vi "Mode 2 - 2D FF AUT Test.vi"() -> (2 "Mode2 Test Properties":T1, 3 "Cancelled?":bool)   [LabVIEW 2019]
doc: "Use this template to create a dialog box with event handling."
uses:
  Mode2TestProperties.ctl
  Classes/Sequence/SequenceSubvis/RF Direction.ctl
panel:
  in  "VNA Calibration File":path
  in  "Number of FF Points":i32
  in  "dPhi (deg)":dbl
  in  "Start Phi (deg)":dbl
  in  "Data File Name":string
  in  "Probe Vertical Polarization":bool
  in  "Probe Horizontal Polarization":bool
  in  "Antenna Tx/Rx":bool
  in  "Upload TR Module file":path=path "C:/Users/Public/Documents/OU PAARD/mmWave_RF_Scanner/SupportFiles/Mode3example1.csv"
  in  "Cancel":bool
  in  "OK":bool
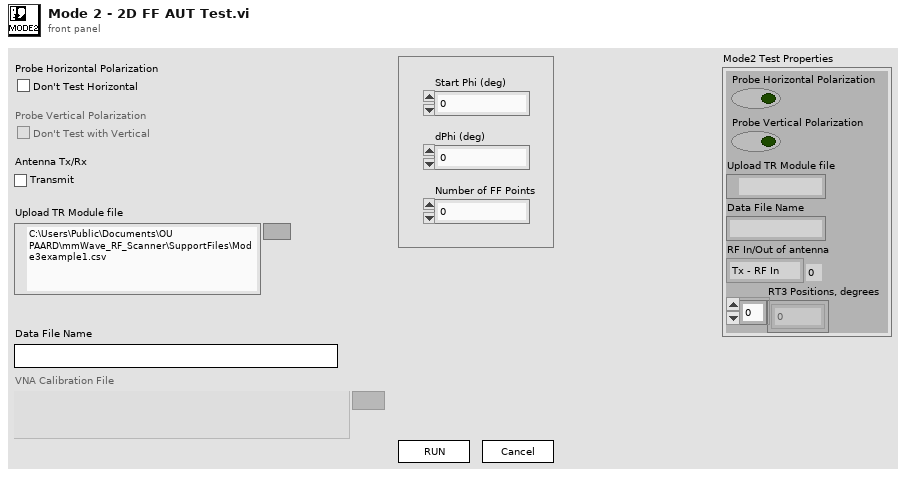
[diagram p1: front panel]
types:
  T1 = typedef "Mode2TestProperties.ctl" = cluster{"Probe Horizontal Polarization":bool, "Probe Vertical Polarization":bool, "Upload TR Module file":path, "Data File Name":string, "RF In/Out of antenna":T2, "RT3 Positions, degrees":dbl[]}
  T2 = typedef "RF Direction.ctl" = enum16{"Tx - RF In", "Rx - RF Out"}
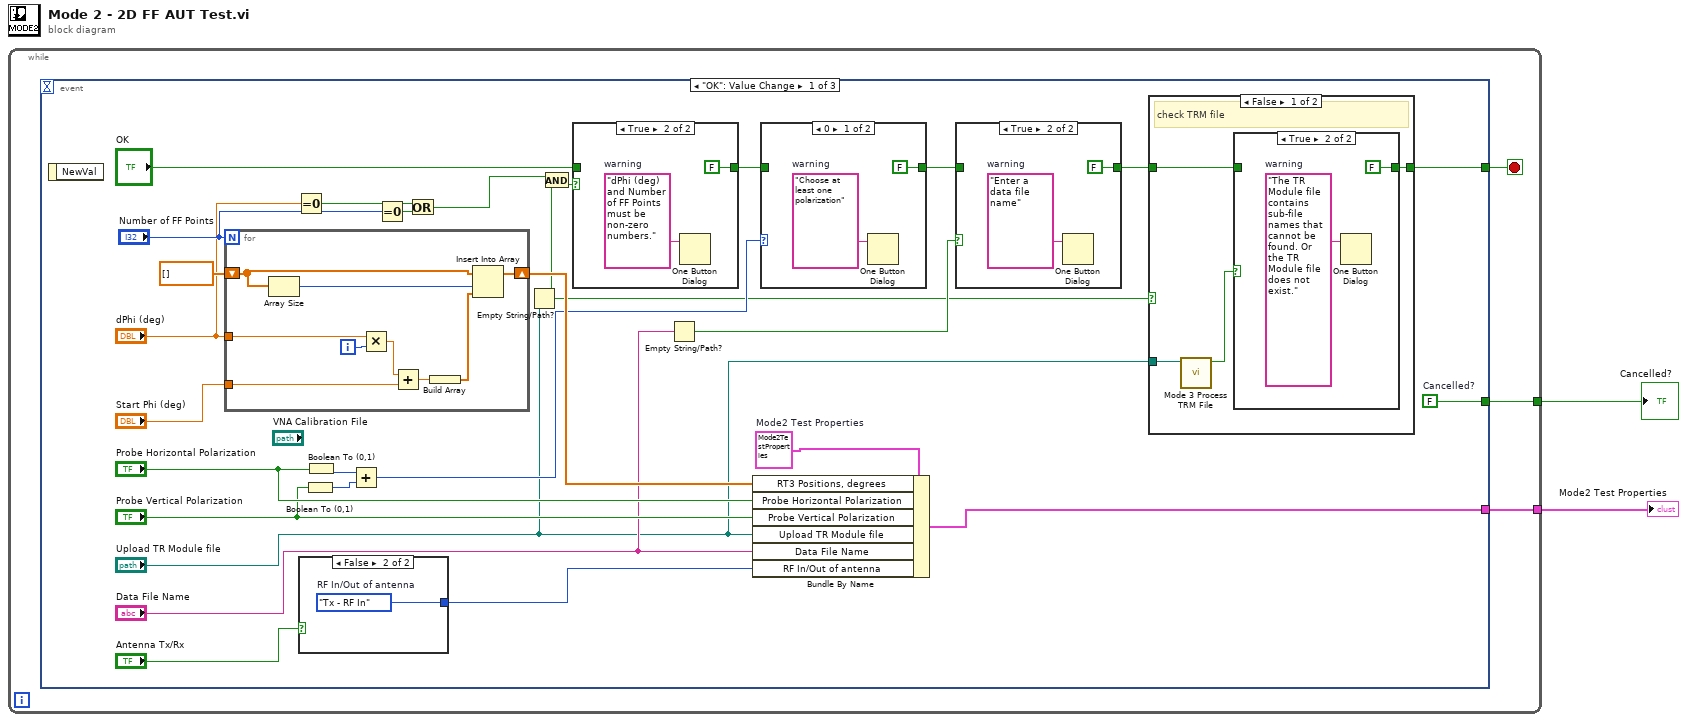
[diagram p0: block diagram]
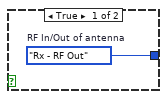
[diagram p7: hidden frame]
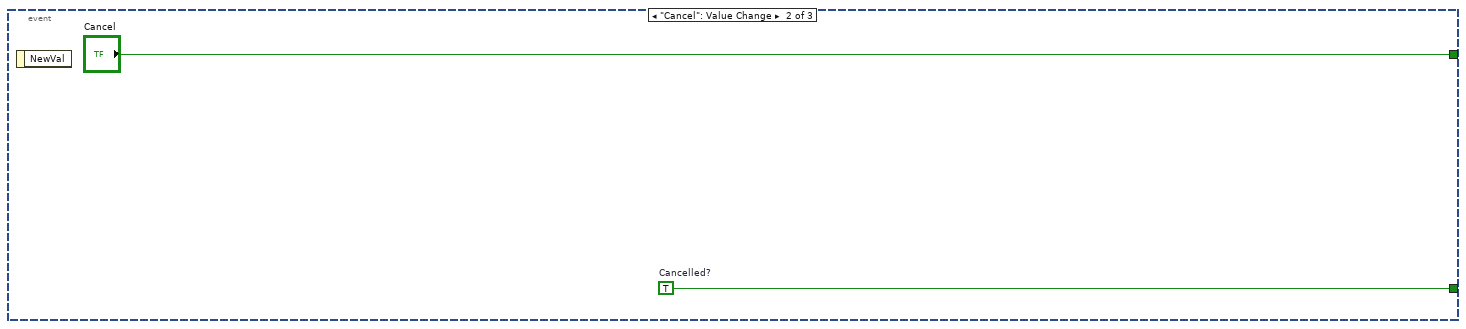
[diagram p8: hidden frame]
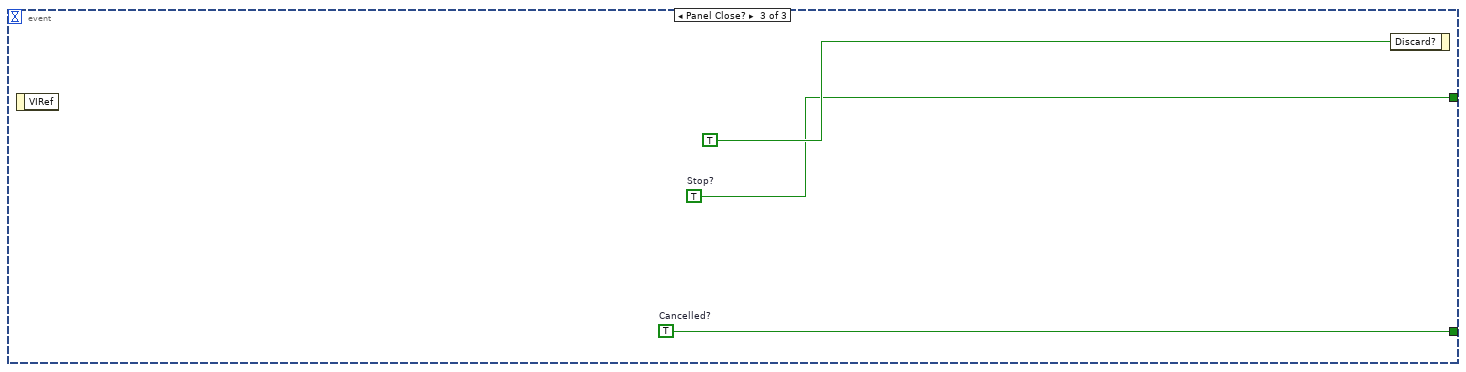
[diagram p9: hidden frame]
diagram:
  n1 = while {
    tunnel: [w4] -> w2
    tunnel: [w3] -> w1
    stop <- w5 stop-if-true
    n2 = event shown="[0] \"OK\": Value Change" {
      selector: _ -> [_ _ _]
      dyn-events: _ -> [_ _ _]
      timeout: _ -> [_ _ _]
      tunnel: [w10 "Cancel" w65] -> w5
      tunnel: [w33 w63 w64] -> w4
      tunnel: [w30 _ _] -> w3
      event "OK": Value Change {
        w29 = T1 {"Probe Horizontal Polarization"=FALSE, "Probe Vertical Polarization"=FALSE, "Upload TR Module file"=path "", "Data File Name"="", "RF In/Out of antenna"=enum."Tx - RF In", "RT3 Positions, degrees"=[]}  # Mode2 Test Properties
        w33 = FALSE  # Cancelled?
        n3 = event-data() -> ()  [unwired: 1 in, 1 out]
        n4 = for {
          N: "Number of FF Points" -> [_]
          shift-right: [w57] -> w27
          shift-left: dbl[] [] -> [w56]
          tunnel: "dPhi (deg)" -> [w52]
          tunnel: "Start Phi (deg)" -> [w51]
          i -> [w59]
          n5 = Array Size(array=w56) -> (size(s)=w53:i32)
          n6 = Multiply(x=w52, y=w59) -> (x*y=w58:dbl)
          n7 = Add(x=w58, y=w51) -> (x+y=w55:dbl)
          n8 = Build Array(w55) -> (w54:dbl[])
          n9 = Insert Into Array(array=w56, index=w53, new element=w54) -> (w57:dbl[])
        }
        n10 = Equal To 0?(x="dPhi (deg)") -> (x = 0?=w23:bool)
        n11 = case shown="False" "Antenna Tx/Rx" {
          tunnel: [w60 w61] -> w31
          frame True {
            w60 = RF_Direction."Rx - RF Out"  # RF In/Out of antenna
          }
          frame False {
            w61 = RF_Direction."Tx - RF In"  # RF In/Out of antenna
          }
        }
        n12 = Boolean To (0,1)(Boolean="Probe Vertical Polarization") -> (0, 1=w18:i16)
        n13 = Boolean To (0,1)(Boolean="Probe Horizontal Polarization") -> (0, 1=w19:i16)
        n14 = Add(x=w19, y=w18) -> (x+y=w16:i16)
        n15 = Equal To 0?(x="Number of FF Points") -> (x = 0?=w25:bool)
        n16 = Or(x=w23, y=w25) -> (x .or. y?=w8:bool)
        n17 = Empty String/Path?(string/path="Upload TR Module file") -> (empty?=w6:bool)
        n18 = And(x=w8, y=w6) -> (x .and. y?=w9:bool)
        n19 = case shown="True" w9 {
          tunnel: [w48 FALSE] -> w17
          tunnel: "OK" -> [w48 _]
          frame False {
          }
          frame True {
            w50 = "dPhi (deg) and Number of FF Points must be non-zero numbers."  # warning
            n20 = One Button Dialog(message=w50) -> ()  [unwired: 1 in, 1 out]
          }
        }
        n21 = Empty String/Path?(string/path="Data File Name") -> (empty?=w13:bool)
        n22 = Bundle By Name(cluster=w29, "RT3 Positions, degrees"=w27, "Probe Horizontal Polarization"="Probe Horizontal Polarization", "Probe Vertical Polarization"="Probe Vertical Polarization", "Upload TR Module file"="Upload TR Module file", "Data File Name"="Data File Name", "RF In/Out of antenna"=w31) -> (w30:T1)
        n23 = case shown="0" w16 {
          tunnel: [FALSE w47] -> w12
          tunnel: w17 -> [_ w47]
          frame 0 {
            w46 = "Choose at least one polarization"  # warning
            n24 = One Button Dialog(message=w46) -> ()  [unwired: 1 in, 1 out]
          }
          frame 1, Default {
          }
        }
        n25 = case shown="True" w13 {
          tunnel: [w42 FALSE] -> w11
          tunnel: w12 -> [w42 _]
          frame False {
          }
          frame True {
            w44 = "Enter a data file name"  # warning
            n26 = One Button Dialog(message=w44) -> ()  [unwired: 1 in, 1 out]
          }
        }
        n27 = case shown="False" w6 {
          tunnel: w11 -> [w36 w41]
          tunnel: [w35 w41] -> w10
          tunnel: "Upload TR Module file" -> [w34 _]
          frame False {
            # "check TRM file"
            n28 = call "Mode 3 Process TRM File.vi"("Upload TR Module file"=w34) -> ("No file = True"=w37:bool)  [unwired: 8 in, 2 out]
            n29 = case shown="True" w37 {
              tunnel: [w38 FALSE] -> w35
              tunnel: w36 -> [w38 _]
              frame False {
              }
              frame True {
                w40 = "The TR Module file contains sub-file names that cannot be found. Or the TR Module file does not exist."  # warning
                n30 = One Button Dialog(message=w40) -> ()  [unwired: 1 in, 1 out]
              }
            }
          }
          frame True {
            # "no file specified"
          }
        }
      }
      event "Cancel": Value Change {
        w63 = TRUE  # Cancelled?
        n31 = event-data() -> ()  [unwired: 1 in, 1 out]
      }
      event Panel Close? {
        w64 = TRUE  # Cancelled?
        w65 = TRUE  # Stop?
        n32 = event-data() -> ()  [unwired: 1 in, 1 out]
        n33 = event-data("Discard?"=TRUE) -> ()  [unwired: 1 in, 1 out]
      }
    }
  }
  "Cancelled?" <- w2
  "Mode2 Test Properties" <- w1
